vi "Cache_Path Global_Read.vi"(5 "Show UI?(F)":bool, 7 "Interrupt":refnum<notifier>, 8 "error in (no error)":errorcluster, 11 "Class Name":string) -> (0 "error out":errorcluster, 1 "Success?":bool, 3 "Class Path":path)   [LabVIEW 2020, in "ClassLoader.lvlib"]
uses:
  ClassLoader.lvlib
  Cache_Path Global.vi
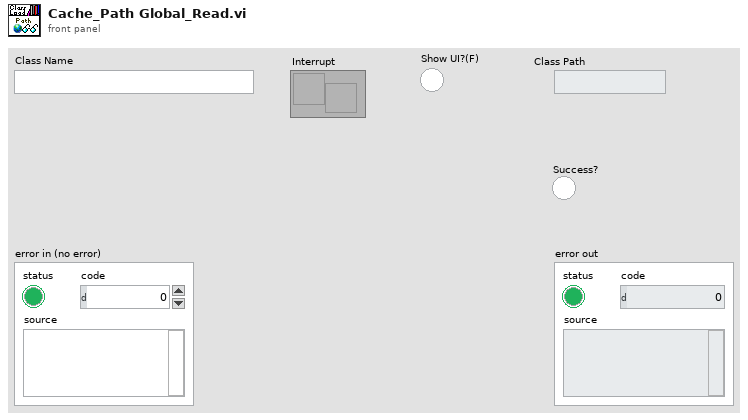
[diagram p1: front panel]
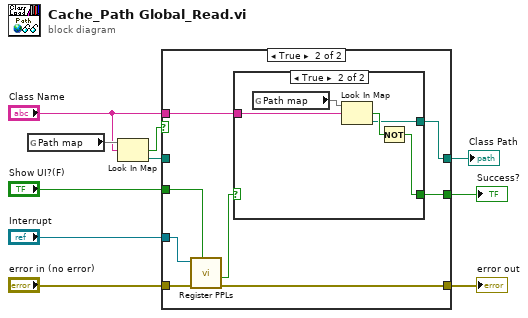
[diagram p0: block diagram]
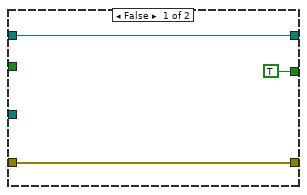
[diagram p2: hidden frame]
diagram:
  n1 = global read "Cache_Path Global.vi" "Path map"() -> (w10:map{string, path})
  n2 = Look In Map(map=w10, key="Class Name") -> (key not found?=w9:bool, value=w6:path)  [unwired: 1 in]
  n3 = case shown="True" w9 {
    tunnel: "error in (no error)" -> [w11 w21]
    tunnel: "Class Name" -> [_ w19]
    tunnel: [w13 w17] -> w5
    tunnel: w6 -> [w13 _]
    tunnel: [TRUE w18] -> w4
    tunnel: [w11 w16] -> w3
    tunnel: "Show UI?(F)" -> [_ w15]
    tunnel: "Interrupt" -> [_ w14]
    frame False {
    }
    frame True {
      n4 = call "Register PPLs.vi"("Show UI?(F)"=w15, "error in"=w21, "Interrupt"=w14) -> ("error out"=w16:errorcluster, "Success?"=w20:bool)  [unwired: 7 in]
      n5 = case shown="True" w20 {
        selector: w20 -> [w22 _]
        tunnel: w19 -> [_ w26]
        tunnel: [w22 w24] -> w18
        tunnel: [_ w23] -> w17
        frame False {
        }
        frame True {
          n6 = global read "Cache_Path Global.vi" "Path map"() -> (w27:map{string, path})
          n7 = Look In Map(map=w27, key=w26) -> (key not found?=w25:bool, value=w23:path)  [unwired: 1 in]
          n8 = Not(x=w25) -> (.not. x?=w24:bool)
        }
      }
    }
  }
  "error out" <- w3
  "Class Path" <- w5
  "Success?" <- w4
